vi "ActionVIOnSave.vi"(8 "error in (no error)":errorcluster, 11 "Device Item Ref in":T1 format="%.0x") -> (0 "error out":errorcluster, 3 "Device Item Ref out":T1 format="%.0x")   [LabVIEW 2017, in "DSF System Explorer.lvlib"]
uses:
  DSF System Explorer.lvlib
  <vilib>/NI Veristand/Custom Device API/Custom Device Item Ref.ctl
  <vilib>/NI Veristand/Custom Device API/Custom Device API.lvlib
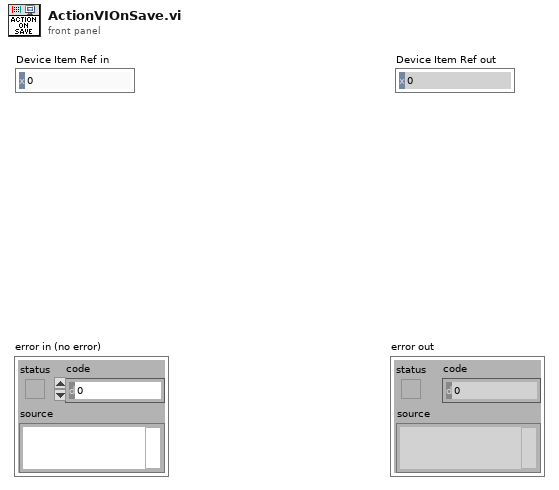
[diagram p1: front panel]
types:
  T1 = typedef "Custom Device API.lvlib/Custom Device Item Ref.ctl" = u64
  T2 = typedef "DSF Core.lvlibp/DSF Engine Framework Configuration.ctl" = cluster{"plugins":T3[]}
  T3 = typedef "DSF Core.lvlibp/DSF Engine Plugin Configuration.ctl" = cluster{"core":T4, "component settings":T6[], "threads":T8[]}
  T4 = typedef "DSF Core.lvlibp/DSF Core Plugin Configuration.ctl" = cluster{"name":string, "components":string[], "cycle timing":T5}
  T5 = typedef "DSF Core.lvlibp/DSF Timing Info.ctl" = cluster{"priority":u64, "decimation":u64, "offset":u64}
  T6 = typedef "DSF Core.lvlibp/DSF Settings Info.ctl" = cluster{"component":string, "version":T7, "values":cluster{"key":string, "value":string}[]}
  T7 = typedef "DSF Core.lvlibp/DSF Version Info.ctl" = cluster{"major":u32, "minor":u32, "fix":u32, "build":string}
  T8 = typedef "DSF Core.lvlibp/DSF Engine Plugin Thread Configuration.ctl" = cluster{"core":T9, "component settings":T6[], "transfer groups":T10[]}
  T9 = typedef "DSF Core.lvlibp/DSF Core Thread Configuration.ctl" = cluster{"processor":i32, "priority offset":i16}
  T10 = typedef "DSF Core.lvlibp/DSF Engine Transfer Group Configuration.ctl" = cluster{"core":T11, "component settings":T6[], "transfers":T14[]}
  T11 = typedef "DSF Core.lvlibp/DSF Core Group Configuration.ctl" = cluster{"name":string, "direction":T12, "cycle timing":T5, "timeout behavior":T13}
  T12 = typedef "DSF Core.lvlibp/DSF Direction.ctl" = enum8{"Tx", "Rx"}
  T13 = typedef "DSF Core.lvlibp/DSF Timeout Behavior.ctl" = enum8{"Increment Late Count", "Throw Error"}
  T14 = typedef "DSF Core.lvlibp/DSF Engine Transfer Configuration.ctl" = cluster{"core":T15, "component settings":T6[], "channels":T16[]}
  T15 = typedef "DSF Core.lvlibp/DSF Core Transfer Configuration.ctl" = cluster{"name":string}
  T16 = typedef "DSF Core.lvlibp/DSF Engine Channel Configuration.ctl" = cluster{"core":T17, "component settings":T6[]}
  T17 = typedef "DSF Core.lvlibp/DSF Core Channel Configuration.ctl" = cluster{"name":string, "units":string, "engine data type":T18, "string data type":T18, "string offset":u64}
  T18 = typedef "DSF Core.lvlibp/DSF Data Type.ctl" = enum8{"Bool", "SGL", "DBL", "I8", "I16", "I32", "I64", "U8", "U16", "U32", "U64"}
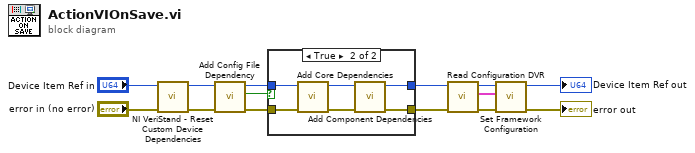
[diagram p0: block diagram]
diagram:
  n1 = call <vilib>:"NI VeriStand - Reset Custom Device Dependencies.vi"("error in (no error)"="error in (no error)", "Device Ref in"="Device Item Ref in") -> ("error out"=w9:errorcluster, "Device Ref out"=w10:T1)  [unwired: 8 in]
  n2 = call "Add Config File Dependency.vi"("error in (no error)"=w9, "Item Ref in"=w10) -> ("error out"=w13:errorcluster, "configuration file set?"=w8:bool, "Device Ref out"=w14:T1)  [unwired: 7 in]
  n3 = case shown="True" w8 {
    tunnel: [w16 w17] -> w7
    tunnel: [w15 w22] -> w6
    tunnel: w14 -> [w16 w19]
    tunnel: w13 -> [w15 w18]
    frame False {
    }
    frame True {
      n4 = call "Add Core Dependencies.vi"("error in (no error)"=w18, "Item Ref in"=w19) -> ("error out"=w20:errorcluster, "Device Ref out"=w21:T1)  [unwired: 8 in]
      n5 = call "Add Component Dependencies.vi"("error in (no error)"=w20, "Device Item Ref in"=w21) -> ("error out"=w22:errorcluster, "Device Ref out"=w17:T1)  [unwired: 7 in, 1 out]
    }
  }
  n6 = call "Read Configuration DVR.vi"("error in (no error)"=w6, "Item Ref in"=w7) -> ("error out"=w4:errorcluster, "framework configuration"=w3:T2, "Item Ref out"=w5:T1)  [unwired: 7 in]
  n7 = call "Set Framework Configuration.vi"("error in (no error)"=w4, "framework configuration"=w3, "Item Ref in"=w5) -> ("error out"=→"error out":errorcluster, "Item Ref out"=→"Device Item Ref out":T1)  [unwired: 7 in]
